vi "Initialise Magnetometer.vi"(8 "error in (no error)":errorcluster, 11 "LSM9DS1 IMU in":refnum<class "LSM9DS1 IMU.lvclass">) -> (0 "error out":errorcluster, 3 "LSM9DS1 IMU out":refnum<class "LSM9DS1 IMU.lvclass">)   [LabVIEW 2020, in "LSM9DS1 IMU.lvclass"]
uses:
  LSM9DS1 IMU.lvclass
  LSM9DS1 IMU.lvclass/LSM9DS1 IMU.ctl
  Read Magnetometer I2C.vi
  Write Magnetometer I2C.vi
  LINX I2C/LINX I2C.lvclass
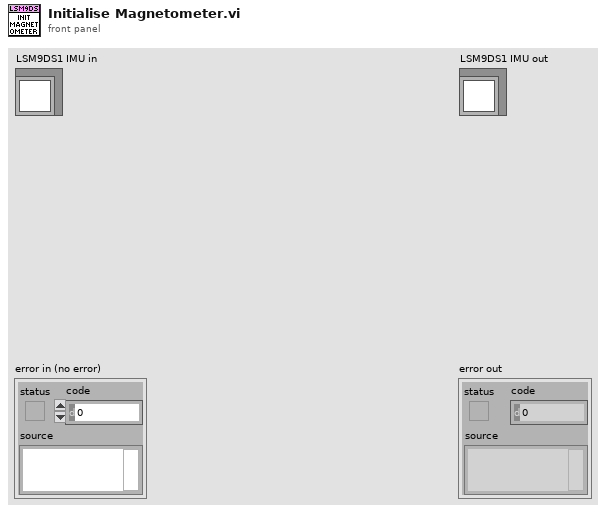
[diagram p1: front panel]
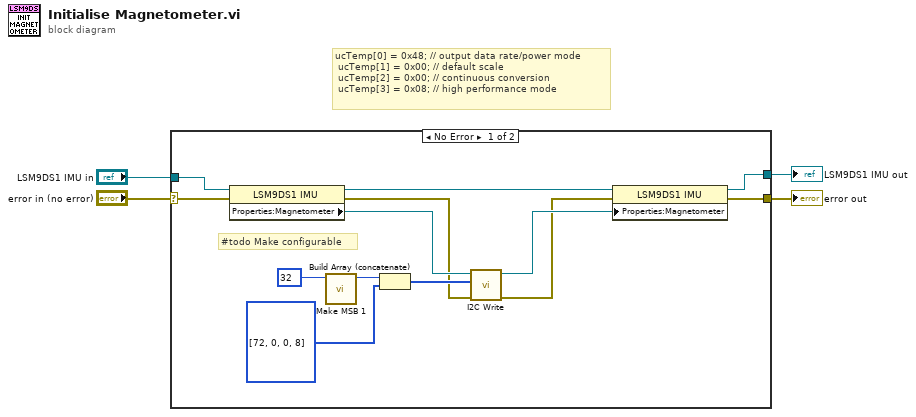
[diagram p0: block diagram]
diagram:
  # "ucTemp[0] = 0x48; // output data rate/power mode\n\tucTemp[1] = 0x00; // default scale\n\tucTemp[2] = 0x00; // continuous conversion\n\tucTemp[3] = 0x08; // high performance mode"
  n1 = case shown="No Error" "error in (no error)" {
    selector: "error in (no error)" -> [w6 w19]
    tunnel: [w5 w19] -> w3
    tunnel: [w14 w18] -> w1
    tunnel: "LSM9DS1 IMU in" -> [w17 w18]
    frame No Error {
      # "#todo Make configurable"
      n2 = property class="LSM9DS1 IMU"(reference=w17, error in=w6) -> (reference out=w15:refnum<class "LSM9DS1 IMU.lvclass">, error out=w8:errorcluster, "Properties:Magnetometer"=w16:refnum<class "LINX I2C.lvclass">)
      n3 = call "Make MSB 1.vi"("Register Address"=u8 32 ("I2C Slave Address 2")) -> ("Register Address | 0x80"=w12:u8)  [unwired: 10 in]
      n4 = Build Array (concatenate)(w12, u8[] [72, 0, 0, 8] ("Bytes to Write")) -> (w10:u8[])
      n5 = call "I2C Write.vi"("error in (no error)"=w8, "Bytes to Write"=w10, "LINX I2C in"=w16) -> ("error out"=w7:errorcluster, "LINX I2C out"=w9:refnum<class "LINX I2C.lvclass">)  [unwired: 7 in]
      n6 = property class="LSM9DS1 IMU"(reference=w15, error in=w7, "Properties:Magnetometer"=w9) -> (reference out=w14:refnum<class "LSM9DS1 IMU.lvclass">, error out=w5:errorcluster)
    }
    frame Error {
    }
  }
  "error out" <- w3
  "LSM9DS1 IMU out" <- w1
